vi "WPI_Dashboard Start Value Logging.vi"(8 "error in (no error)":errorcluster) -> (0 "error out":errorcluster, 1 "handles":cluster{"poller":u32, "overAll Listener":u32})   [LabVIEW 2025]
uses:
  ntcoreffi.dll
  FRC_NetworkTablesLV.dll
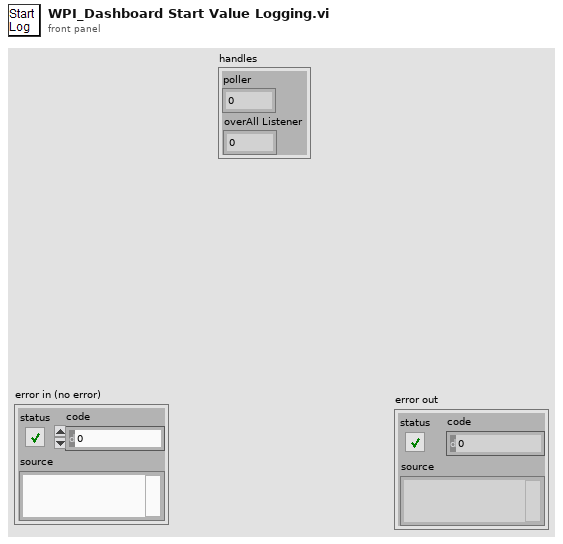
[diagram p1: front panel]
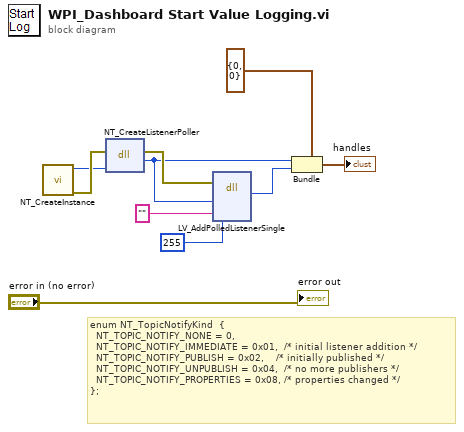
[diagram p0: block diagram]
diagram:
  # "enum NT_TopicNotifyKind\t {\n  NT_TOPIC_NOTIFY_NONE = 0,\n  NT_TOPIC_NOTIFY_IMMEDIATE = 0x01,  /* initial listener addition */\n  NT_TOPIC_NOTIFY_PUBLISH = 0x02,    /* initially published */\n  NT_TOPIC_NOTIFY_UNPUBLISH = 0x04,  /* no more publishers */\n  NT_TOPIC_NOTIFY_PROPERTIES = 0x08, /* properties changed */\n};"
  n1 = call <vilib>:"NT_CreateInstance.vi"() -> ("error out"=w10:errorcluster, "InstanceHandle"=w9:u64)  [unwired: 10 in]
  n2 = dll-call lib="ntcoreffi.*" fn="NT_CreateListenerPoller"(error in=w10, "inst"=w9) -> (error out=w3:errorcluster, "poller"=w2:u32)  [unwired: 3 in, 1 out]
  n3 = dll-call lib="FRC_NetworkTablesLV.*" fn="LV_AddPolledListenerSingle"(error in=w3, "poller"=w2, "prefix"="", "mask"=u32 255) -> ("topicListener"=w1:u32)  [unwired: 5 in, 2 out]
  n4 = Bundle(cluster=cluster{"valuePoller":u32, "topicListener":u32} {"valuePoller"=0, "topicListener"=0} ("handles"), "valuePoller"=w2, "topicListener"=w1) -> (→"handles":cluster{"valuePoller":u32, "topicListener":u32})
  "error out" <- "error in (no error)"
